vi "SetTemperature.vi"(8 "error in (no error)":errorcluster, 10 "Temperature (°C)":dbl min=0.0 max=450.0 step=1.0, 11 "VISA Refnum in":refnum<visa-resource-name>) -> (0 "error in (no error) 2":errorcluster, 3 "VISA Refnum Out":refnum<visa-resource-name>)   [LabVIEW 2023]
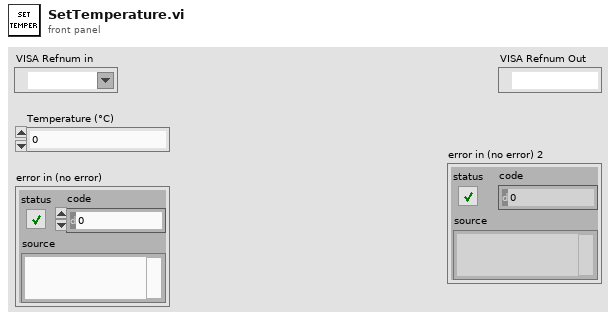
[diagram p1: front panel]
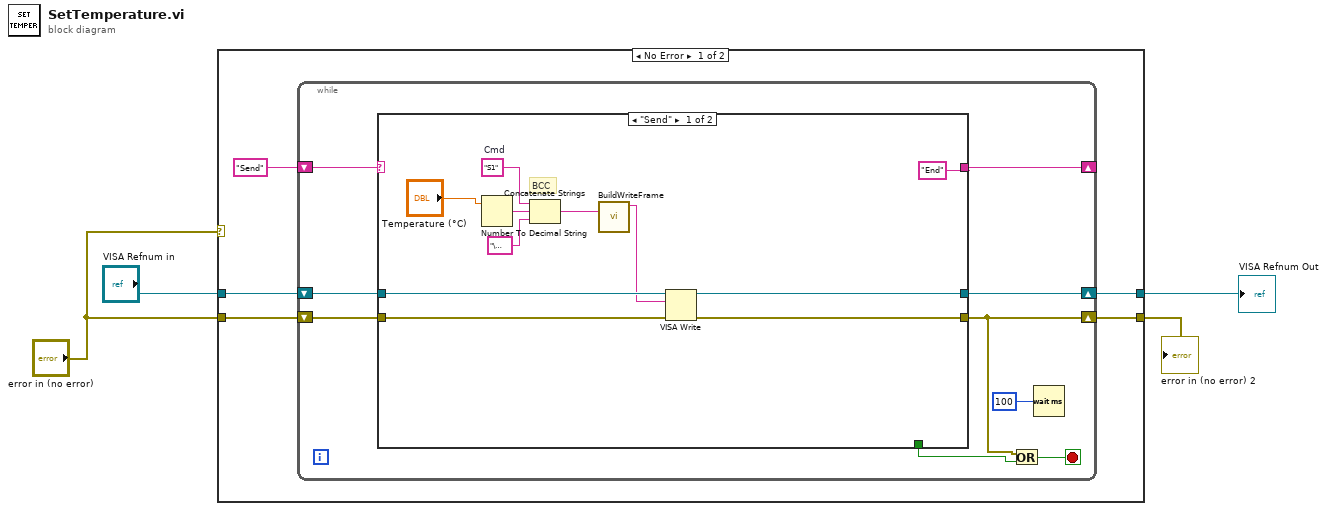
[diagram p0: block diagram]
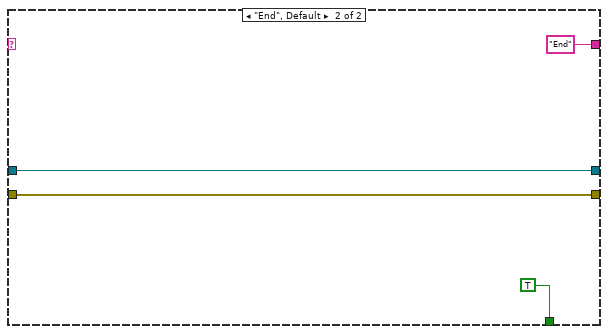
[diagram p2: hidden frame]
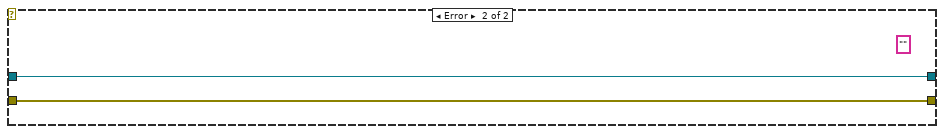
[diagram p3: hidden frame]
diagram:
  n1 = case shown="No Error" "error in (no error)" {
    tunnel: "VISA Refnum in" -> [w9 w35]
    tunnel: "error in (no error)" -> [w8 w34]
    tunnel: [w6 w35] -> w1
    tunnel: [w5 w34] -> w2
    frame No Error {
      n2 = while {
        shift-right: [w15] -> _
        shift-left: "Send" -> [w16]
        shift-right: [w10] -> w6
        shift-left: w9 -> [w18]
        shift-right: [w11] -> w5
        shift-left: w8 -> [w17]
        stop <- w13 stop-if-true
        n3 = case shown="\"Send\"" w16 {
          tunnel: w18 -> [w29 w31]
          tunnel: w17 -> [w28 w32]
          tunnel: ["End" "End"] -> w15
          tunnel: [_ TRUE] -> w12
          tunnel: [w26 w32] -> w11
          tunnel: [w25 w31] -> w10
          frame "Send" {
            w24 = "S1"  # Cmd
            # "BCC"
            n4 = Number To Decimal String(number="Temperature (°C)") -> (decimal integer string=w23:string)  [unwired: 1 in]
            n5 = Concatenate Strings(w24, w23, "\u0003" ("string")) -> (w21:string)
            n6 = call "BuildWriteFrame.vi"("String in"=w21) -> ("String out"=w20:string)  [unwired: 10 in]
            n7 = VISA Write(VISA resource name=w29, write buffer=w20, error in (no error)=w28) -> (VISA resource name out=w25:refnum<visa-resource-name>, error out=w26:errorcluster)  [unwired: 1 out]
          }
          frame "End", Default {
          }
        }
        n8 = Or(x=w11, y=w12) -> (x .or. y?=w13:bool)
        n9 = Wait (ms)(milliseconds to wait=u32 100) -> ()  [unwired: 1 out]
      }
    }
    frame Error {
      (unwired) "" ("read buffer")
    }
  }
  "VISA Refnum Out" <- w1
  "error in (no error) 2" <- w2
